vi "ConvertGoop2ToGoop3_RecompileAll.vi"(6 "error IO 2":errorcluster, 7 "VIsToRelink":refnum<vi>[](array[refnum]), 8 "Classes":T1[](array[typedef]), 9 "Cluster 2":T6) -> (0 "error IO":errorcluster)   [LabVIEW 2020]
uses:
  ConvertGoop2ToGoop3_ClassInfo.ctl
  LvClass_class/GDSLvCLass_ClassSettingsType.ctl
  LvClass_class/GDSLvClass_PlugIn.ctl
  LvClass_class/GDSLvClass_PlugInTypes.ctl
  <vilib>/Utility/miscctls.llb/LVPositionTypeDef.ctl
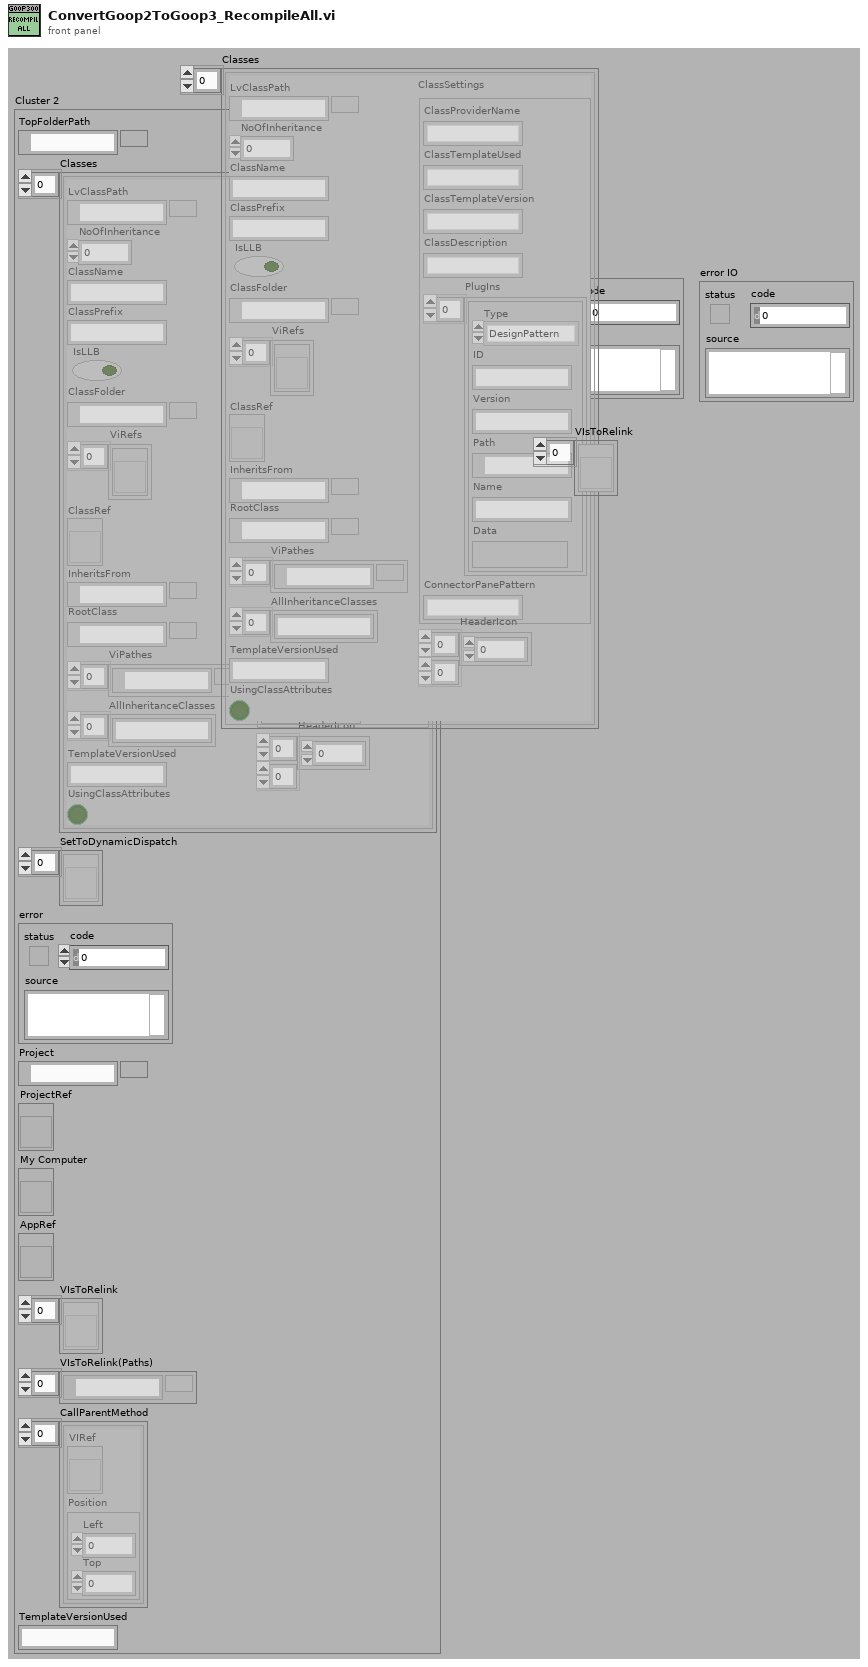
[diagram p1: front panel]
types:
  T1 = typedef "ConvertGoop2ToGoop3_ClassInfo.ctl" = cluster{"NoOfInheritance":i32, "LvClassPath":path, "ClassName":string, "ClassPrefix":string, "IsLLB":bool, "ClassFolder":path, "ViRefs":refnum<vi>[], "ClassRef":refnum<vi>, "InheritsFrom":path, "RootClass":path, "ViPathes":path[], "AllInheritanceClasses":string[], "TemplateVersionUsed":string, "UsingClassAttributes":bool, "ClassSettings":T2, "HeaderIcon":u8[][]}
  T2 = typedef "GDSLvCLass_ClassSettingsType.ctl" = cluster{"ClassProviderName":string, "ClassTemplateUsed":string, "ClassTemplateVersion":string, "ClassDescription":string, "PlugIns":T3[], "ConnectorPanePattern":string}
  T3 = typedef "GDSLvClass_PlugIn.ctl" = cluster{"Type":T4, "ID":string, "Version":string, "Path":path, "Name":string, "Data":variant}
  T4 = typedef "GDSLvClass_PlugInTypes.ctl" = enum16{"DesignPattern", "MethodTypes"}
  T5 = typedef "LVPositionTypeDef.ctl" = cluster{"Left":i32, "Top":i32}
  T6 = cluster{"TopFolderPath":path, "Classes":T1[], "SetToDynamicDispatch":refnum<vi>[], "error":errorcluster, "Project":path, "ProjectRef":refnum<vi>, "My Computer":refnum<vi>, "AppRef":refnum<vi>, "VIsToRelink":refnum<vi>[], "VIsToRelink(Paths)":path[], "CallParentMethod":cluster{"VIRef":refnum<vi>, "Position":T5}[], "TemplateVersionUsed":string}
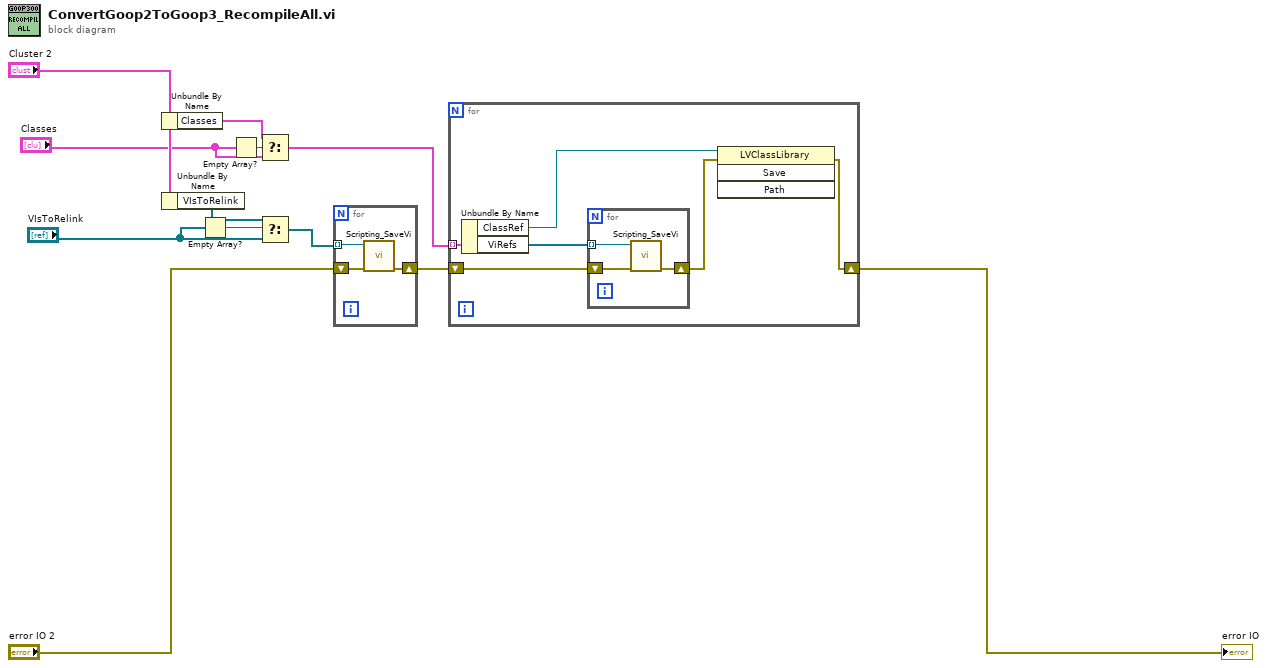
[diagram p0: block diagram]
diagram:
  n1 = Unbundle By Name("Cluster 2") -> ("Classes"=w6:T1[])
  n2 = Unbundle By Name("Cluster 2") -> ("VIsToRelink"=w4:refnum<vi>[])
  n3 = Empty Array?(array="VIsToRelink") -> (empty?=w1:bool)
  n4 = Empty Array?(array="Classes") -> (empty?=w8:bool)
  n5 = Select(t=w6, s=w8, f="Classes") -> (s? t:f=w5:T1[])
  n6 = Select(t=w4, s=w1, f="VIsToRelink") -> (s? t:f=w3:refnum<vi>[])
  n7 = for {
    tunnel: w3 -> [w15] mode=indexing
    shift-right: [w13] -> w11
    shift-left: "error IO 2" -> [w14]
    n8 = call "Scripting_SaveVi.vi"("error in (no error)"=w14, "VIRefToSaveIn"=w15) -> ("error out"=w13:errorcluster)  [unwired: 8 in, 1 out]
  }
  n9 = for {
    tunnel: w5 -> [w20] mode=indexing
    shift-right: [w16] -> w12
    shift-left: w11 -> [w21]
    n10 = Unbundle By Name(w20) -> ("ClassRef"=w18:refnum<vi>, "ViRefs"=w19:refnum<vi>[])
    n11 = for {
      tunnel: w19 -> [w22] mode=indexing
      shift-right: [w23] -> w17
      shift-left: w21 -> [w24]
      n12 = call "Scripting_SaveVi.vi"("error in (no error)"=w24, "VIRefToSaveIn"=w22) -> ("error out"=w23:errorcluster)  [unwired: 8 in, 1 out]
    }
    n13 = invoke class="LVClassLibrary" method="Save"(reference=w18, error in=w17) -> (error out=w16:errorcluster)  [unwired: 2 in, 3 out]
  }
  "error IO" <- w12
